vi "_VI Visible.vi"(8 "error in (no error)":errorcluster, 11 "VI in":refnum<vi>) -> (0 "error out":errorcluster, 2 "visible":bool, 3 "VI out":refnum<vi>)   [LabVIEW 2014, in "UI_ProgressDlg.lvlib" / "UI_ProgressDlg.lvclass"]
uses:
  UI_ProgressDlg.lvclass
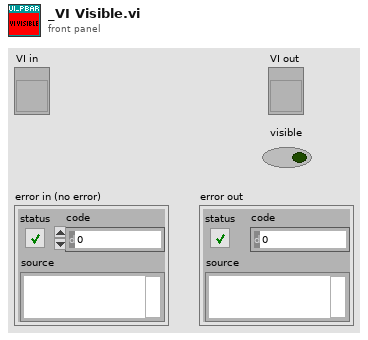
[diagram p1: front panel]
types:
  T1 = enum32{"Invalid", "Standard", "Closed", "Hidden", "Minimized", "Maximized"}
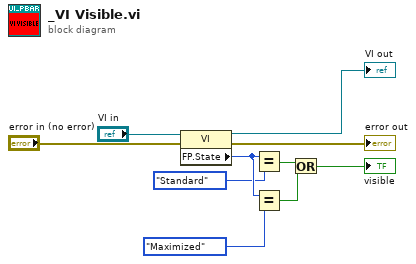
[diagram p0: block diagram]
diagram:
  n1 = property on="Property Node" class="VI"(reference="VI in", error in="error in (no error)") -> (reference out=→"VI out":refnum<vi>, error out=→"error out":errorcluster, "FP.State"=w6:T1)
  n2 = Equal?(x=w6, y=T1."Standard") -> (x = y?=w7:bool)
  n3 = Equal?(x=w6, y=T1."Maximized") -> (x = y?=w8:bool)
  n4 = Or(x=w7, y=w8) -> (x .or. y?=→"visible":bool)
